vi "UsingTheToolsPalette.vi"() -> ()   [LabVIEW 2018]
panel:
  in  "stop":bool
  out "LED":bool
  in  "Toggle":bool
  out "Thermometer":dbl(slide) scale=0.0..100.0
  in  "Slide":dbl(slide) scale=0.0..100.0
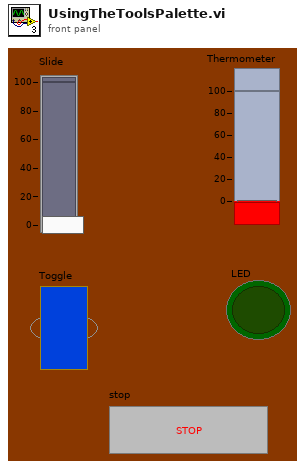
[diagram p1: front panel]
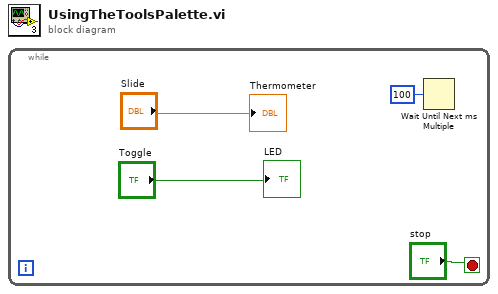
[diagram p0: block diagram]
diagram:
  n1 = while {
    stop <- "stop" stop-if-true
    n2 = Wait Until Next ms Multiple(millisecond multiple=u32 100) -> ()  [unwired: 1 out]
    "Thermometer" <- "Slide"
    "LED" <- "Toggle"
  }
